vi "Set Elevator Height.vi"(10 "Height":dbl, 11 "Execute?":bool) -> (3 "Done":bool)   [LabVIEW 2012]
uses:
  Globals/Useful Values.vi
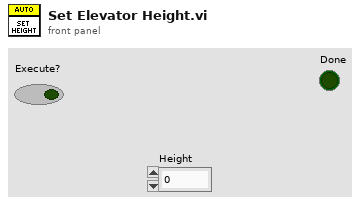
[diagram p1: front panel]
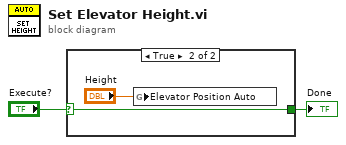
[diagram p0: block diagram]
diagram:
  n1 = case shown="True" "Execute?" {
    selector: "Execute?" -> [w3 w5]
    tunnel: [w3 w5] -> w1
    frame False {
    }
    frame True {
      n2 = global write "Useful Values.vi" "Elevator Position Auto"("Height") -> ()
    }
  }
  "Done" <- w1
